vi "Parse Readings Value TST.vi"(11 "Readings":string) -> (0 "count":dbl format="%#_13g", 1 "Time":dbl format="%#_13g", 2 "Measurement":dbl format="%#_13g", 3 "Remain Readings":string)   [LabVIEW 2016, in "ElectrometerController.lvclass"]
doc: "Parse the readings according to format."
uses:
  ElectrometerController/ElectrometerController.lvclass
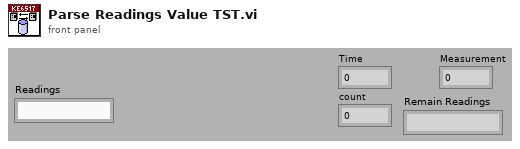
[diagram p1: front panel]
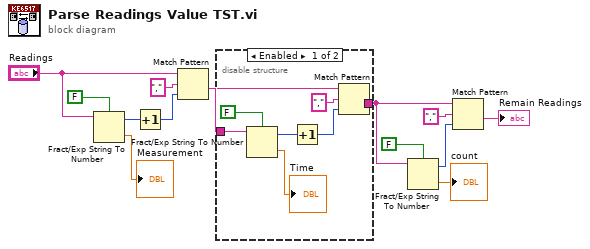
[diagram p0: block diagram]
diagram:
  n1 = Fract/Exp String To Number(use system decimal point (T)=FALSE, string="Readings") -> (offset past number=w8:i32, number=→"Measurement":dbl)  [unwired: 2 in]
  n2 = Increment(x=w8) -> (x+1=w12:i32)
  n3 = Match Pattern(string="Readings", regular expression=",", offset (0)=w12) -> (after substring=w7:string)  [unwired: 3 out]
  n4 = disable-structure shown="Enabled" {
    disable-tunnel: w7 -> [w15 w21]
    disable-tunnel: [w14 w21] -> w3
    frame Enabled {
      n5 = Fract/Exp String To Number(use system decimal point (T)=FALSE, string=w15) -> (offset past number=w18:i32, number=→"Time":dbl)  [unwired: 2 in]
      n6 = Increment(x=w18) -> (x+1=w17:i32)
      n7 = Match Pattern(string=w15, regular expression=",", offset (0)=w17) -> (after substring=w14:string)  [unwired: 3 out]
    }
    frame Disabled {
    }
  }
  n8 = Fract/Exp String To Number(use system decimal point (T)=FALSE, string=w3) -> (offset past number=w4:i32, number=→"count":dbl)  [unwired: 2 in]
  n9 = Match Pattern(string=w3, regular expression=",", offset (0)=w4) -> (after substring=→"Remain Readings":string)  [unwired: 3 out]
